vi "Propeller_setup.vi"(1 "Setup String":string) -> (0 "Output string":string)   [LabVIEW 2010]
uses:
  Controls/ok_button.ctl
panel:
  in  "OK":T1
  in  "Propeller anemometer setup":cluster{"Probe type":u16, "Anemometer box":u16} {"Anemometer box" items=["Mini Air 2", "Mini Air 5"]; "Probe type" items=["624.24", "662/51"]}
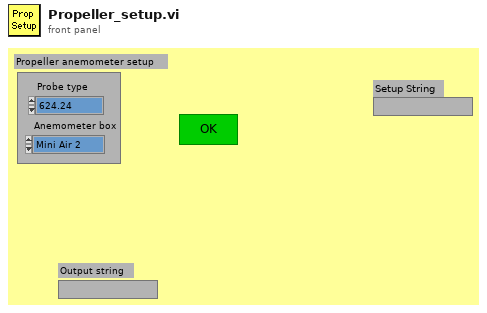
[diagram p1: front panel]
types:
  T1 = typedef "ok_button.ctl" = bool
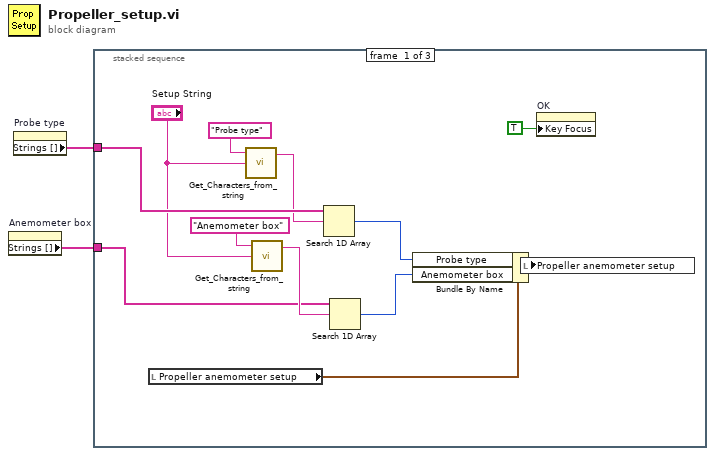
[diagram p0: block diagram]
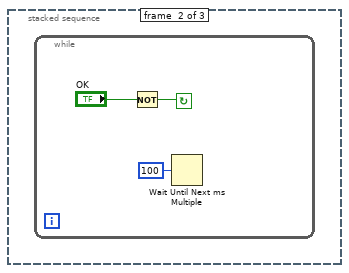
[diagram p2: hidden frame]
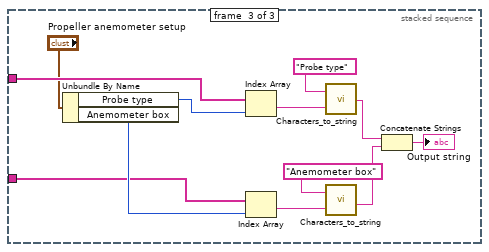
[diagram p3: hidden frame]
diagram:
  n1 = property on="Anemometer box" class="Ring (strict)"() -> ("Strings []"=w1:string[])  [unwired: 2 in, 2 out]
  n2 = property on="Probe type" class="Ring (strict)"() -> ("Strings []"=w2:string[])  [unwired: 2 in, 2 out]
  n3 = stacked-sequence {
    tunnel: w2 -> [w11 _ w20]
    tunnel: w1 -> [w6 _ w19]
    frame #0 {
      n4 = local read "Propeller anemometer setup"() -> (w14:cluster{"Probe type":u16, "Anemometer box":u16})
      n5 = call "Get_Characters_from_string.vi"("Input string"="Setup String", "Variable name"="Probe type") -> ("Value"=w10:string)  [unwired: 1 in, 1 out]
      n6 = call "Get_Characters_from_string.vi"("Input string"="Setup String", "Variable name"="Anemometer box") -> ("Value"=w8:string)  [unwired: 1 in, 1 out]
      n7 = Search 1D Array(1D array=w11, element=w10) -> (index of element=w9:i32)  [unwired: 1 out]
      n8 = Search 1D Array(1D array=w6, element=w8) -> (index of element=w4:i32)  [unwired: 1 out]
      n9 = Bundle By Name(cluster=w14, "Probe type"=w9, "Anemometer box"=w4) -> (w13:cluster{"Probe type":u16, "Anemometer box":u16})
      n10 = local write "Propeller anemometer setup"(w13) -> ()
      n11 = property on="OK" class="Bool"("Key Focus"=TRUE) -> ()  [unwired: 2 in, 2 out]
    }
    frame #1 {
      n12 = while {
        stop <- w17 continue-if-true
        n13 = Not(x="OK") -> (.not. x?=w17:T1)
        n14 = Wait Until Next ms Multiple(millisecond multiple=u32 100) -> ()  [unwired: 1 out]
      }
    }
    frame #2 {
      n15 = Unbundle By Name("Propeller anemometer setup") -> ("Probe type"=w22:u16, "Anemometer box"=w21:u16)
      n16 = Index Array(array=w20, index=w22) -> (element=w25:string)
      n17 = Index Array(array=w19, index=w21) -> (element=w23:string)
      n18 = call "Characters_to_string.vi"("Characters to write"=w25, "Label for characters"="Probe type") -> ("Output string"=w27:string)
      n19 = call "Characters_to_string.vi"("Characters to write"=w23, "Label for characters"="Anemometer box") -> ("Output string"=w28:string)
      n20 = Concatenate Strings(w27, w28) -> (→"Output string":string)
    }
  }
